vi "subvi_string_to_serial_message.vi"(6 "Type":enum16{"ReadableChars", "SpellmanMPS"}(ring), 10 "Input Message":string) -> (2 "Serial Message":string)   [LabVIEW 2014]
doc: "Input is a string which the user wants to send over serial. \nThe output is that string message + a checksum of the Type + a linefeed."
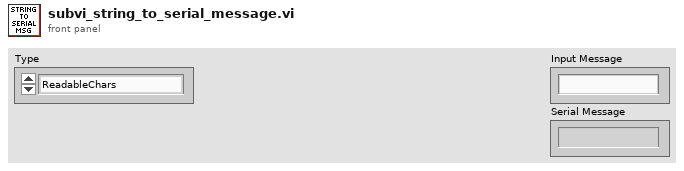
[diagram p1: front panel]
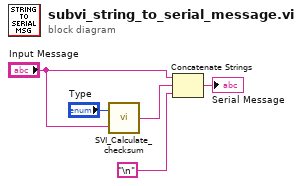
[diagram p0: block diagram]
diagram:
  n1 = call "SVI_Calculate_checksum.vi"("Message"="Input Message", "Type"="Type") -> ("Calculated checksum"=w4:string)
  n2 = Concatenate Strings("Input Message", w4, "\n") -> (→"Serial Message":string)
